vi "Day 16-Get Substring.vi"(10 "length":i32=3, 11 "String in":string) -> (2 "Substring":string, 3 "String out":string)   [LabVIEW 2021]
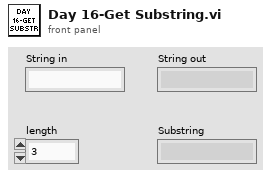
[diagram p1: front panel]
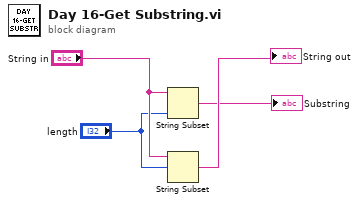
[diagram p0: block diagram]
diagram:
  n1 = String Subset(string="String in", length (rest)="length") -> (substring=→"Substring":string)  [unwired: 1 in]
  n2 = String Subset(string="String in", offset (0)="length") -> (substring=→"String out":string)  [unwired: 1 in]
